vi "ArmRecoverHomePosition.vi"(0 "ArmRecoveryParameters In":T23, 1 "ArmRecoveryOffsets":T24, 2 "RobotConfig":T2={"Motors"={"DriveRightPrimary"={"CAN Address"=1, "Invert"=FALSE, "InvertSensor"=FALSE, "Unit Conversion Factor"=0.0, "Brake Mode"=enum."Override to Brake", "Reverse Limt Switch Mode"=enum."Normally Closed", "Forward Limt Swith Mode"=enum."Normally Closed", "PWM Channel"=enum."Invalid", "Motor Controller Type"=enum."Talon SRX", "Peak Current (A)"=0, "Continuos Current (A)"=0, "Peak Duration (ms)"=0, "Current Limit Enable"=FALSE}, "DriveRightSecondary"={"CAN Address"=2, "Invert"=FALSE, "InvertSensor"=FALSE, "Unit Conversion Factor"=0.0, "Brake Mode"=enum."Override to Brake", "Reverse Limt Switch Mode"=enum."Normally Closed", "Forward Limt Swith Mode"=enum."Normally Closed", "PWM Channel"=enum."Invalid", "Motor Controller Type"=enum."Talon SRX", "Peak Current (A)"=0, "Continuos Current (A)"=0, "Peak Duration (ms)"=0, "Current Limit Enable"=FALSE}, "DriveLeftPrimary"={"CAN Address"=3, "Invert"=FALSE, "InvertSensor"=FALSE, "Unit Conversion Factor"=0.0, "Brake Mode"=enum."Override to Brake", "Reverse Limt Switch Mode"=enum."Normally Closed", "Forward Limt Swith Mode"=enum."Normally Closed", "PWM Channel"=enum."Invalid", "Motor Controller Type"=enum."Talon SRX", "Peak Current (A)"=0, "Continuos Current (A)"=0, "Peak Duration (ms)"=0, "Current Limit Enable"=FALSE}, "DriveLeftSecondary"={"CAN Address"=4, "Invert"=FALSE, "InvertSensor"=FALSE, "Unit Conversion Factor"=0.0, "Brake Mode"=enum."Override to Brake", "Reverse Limt Switch Mode"=enum."Normally Closed", "Forward Limt Swith Mode"=enum."Normally Closed", "PWM Channel"=enum."Invalid", "Motor Controller Type"=enum."Talon SRX", "Peak Current (A)"=0, "Continuos Current (A)"=0, "Peak Duration (ms)"=0, "Current Limit Enable"=FALSE}, "RearClimb"={"CAN Address"=8, "Invert"=FALSE, "InvertSensor"=FALSE, "Unit Conversion Factor"=0.0, "Brake Mode"=enum."Override to Brake", "Reverse Limt Switch Mode"=enum."Normally Closed", "Forward Limt Swith Mode"=enum."Normally Closed", "PWM Channel"=enum."Invalid", "Motor Controller Type"=enum."Talon SRX", "Peak Current (A)"=0, "Continuos Current (A)"=0, "Peak Duration (ms)"=0, "Current Limit Enable"=FALSE}, "Front Climb"={"CAN Address"=7, "Invert"=FALSE, "InvertSensor"=FALSE, "Unit Conversion Factor"=0.0, "Brake Mode"=enum."Override to Brake", "Reverse Limt Switch Mode"=enum."Normally Closed", "Forward Limt Swith Mode"=enum."Normally Closed", "PWM Channel"=enum."Invalid", "Motor Controller Type"=enum."Talon SRX", "Peak Current (A)"=0, "Continuos Current (A)"=0, "Peak Duration (ms)"=0, "Current Limit Enable"=FALSE}, "Climb Drive"={"CAN Address"=5, "Invert"=FALSE, "InvertSensor"=FALSE, "Unit Conversion Factor"=0.0, "Brake Mode"=enum."Override to Brake", "Reverse Limt Switch Mode"=enum."Normally Closed", "Forward Limt Swith Mode"=enum."Normally Closed", "PWM Channel"=enum."Invalid", "Motor Controller Type"=enum."Talon SRX", "Peak Current (A)"=0, "Continuos Current (A)"=0, "Peak Duration (ms)"=0, "Current Limit Enable"=FALSE}, "Shoulder1"={"CAN Address"=6, "Invert"=FALSE, "InvertSensor"=FALSE, "Unit Conversion Factor"=0.0, "Brake Mode"=enum."Override to Brake", "Reverse Limt Switch Mode"=enum."Normally Closed", "Forward Limt Swith Mode"=enum."Normally Closed", "PWM Channel"=enum."Invalid", "Motor Controller Type"=enum."Talon SRX", "Peak Current (A)"=0, "Continuos Current (A)"=0, "Peak Duration (ms)"=0, "Current Limit Enable"=FALSE}, "Shoulder2"={"CAN Address"=9, "Invert"=FALSE, "InvertSensor"=FALSE, "Unit Conversion Factor"=0.0, "Brake Mode"=enum."Override to Brake", "Reverse Limt Switch Mode"=enum."Normally Closed", "Forward Limt Swith Mode"=enum."Normally Closed", "PWM Channel"=enum."Invalid", "Motor Controller Type"=enum."Talon SRX", "Peak Current (A)"=0, "Continuos Current (A)"=0, "Peak Duration (ms)"=0, "Current Limit Enable"=FALSE}, "Wrist"={"CAN Address"=10, "Invert"=FALSE, "InvertSensor"=FALSE, "Unit Conversion Factor"=0.0, "Brake Mode"=enum."Override to Brake", "Reverse Limt Switch Mode"=enum."Disabled", "Forward Limt Swith Mode"=enum."Disabled", "PWM Channel"=enum."Invalid", "Motor Controller Type"=enum."Talon SRX", "Peak Current (A)"=0, "Continuos Current (A)"=0, "Peak Duration (ms)"=0, "Current Limit Enable"=FALSE}, "Extension"={"CAN Address"=11, "Invert"=FALSE, "InvertSensor"=FALSE, "Unit Conversion Factor"=0.0, "Brake Mode"=enum."Override to Brake", "Reverse Limt Switch Mode"=enum."Disabled", "Forward Limt Swith Mode"=enum."Disabled", "PWM Channel"=enum."Invalid", "Motor Controller Type"=enum."Talon SRX", "Peak Current (A)"=0, "Continuos Current (A)"=0, "Peak Duration (ms)"=0, "Current Limit Enable"=FALSE}, "CargoIntake"={"CAN Address"=11, "Invert"=FALSE, "InvertSensor"=FALSE, "Unit Conversion Factor"=0.0, "Brake Mode"=enum."Override to Brake", "Reverse Limt Switch Mode"=enum."Disabled", "Forward Limt Swith Mode"=enum."Disabled", "PWM Channel"=enum."Invalid", "Motor Controller Type"=enum."Talon SRX", "Peak Current (A)"=0, "Continuos Current (A)"=0, "Peak Duration (ms)"=0, "Current Limit Enable"=FALSE}, "Intake2"={"CAN Address"=11, "Invert"=FALSE, "InvertSensor"=FALSE, "Unit Conversion Factor"=0.0, "Brake Mode"=enum."Override to Brake", "Reverse Limt Switch Mode"=enum."Disabled", "Forward Limt Swith Mode"=enum."Disabled", "PWM Channel"=enum."Invalid", "Motor Controller Type"=enum."Talon SRX", "Peak Current (A)"=0, "Continuos Current (A)"=0, "Peak Duration (ms)"=0, "Current Limit Enable"=FALSE}}, "Sensors"={"IMU"={"Yaw Axis"=enum."Z", "SPI Bus"=enum."SPI MXP", "AHRS Algorithm"=enum."Complementary", "Calibration Time (s)"=3.0, "Calibrate On Open"=TRUE}, "HomingButton"={"DIOChannel"=enum."DIO 0", "Active Low"=FALSE}, "HomingLED_Green"={"DIOChannel"=enum."DIO 0", "Active Low"=FALSE}, "HomingLED_Yellow"={"DIOChannel"=enum."DIO 0", "Active Low"=FALSE}, "HomingLED_Red"={"DIOChannel"=enum."DIO 0", "Active Low"=FALSE}}, "PID"={"FrontClimb"={"P"=0.0, "I"=0.0, "D"=0.0, "F"=0.0, "IZone"=0.0}, "RearClimb"={"P"=0.0, "I"=0.0, "D"=0.0, "F"=0.0, "IZone"=0.0}, "ArmShoulder"={"P"=0.0, "I"=0.0, "D"=0.0, "F"=0.0, "IZone"=0.0}, "ArmExtend"={"P"=0.0, "I"=0.0, "D"=0.0, "F"=0.0, "IZone"=0.0}, "ArmWrist"={"P"=0.0, "I"=0.0, "D"=0.0, "F"=0.0, "IZone"=0.0}}, "Solenoids"={" Shifter"={"SolenoidChannel"=enum."Solenoid 3", "Invert"=FALSE}, "Hatch Grip"={"SolenoidChannel"=enum."Solenoid 0", "Invert"=FALSE}, "Hatch Extend"={"SolenoidChannel"=enum."Solenoid 0", "Invert"=FALSE}, "Manipulator Slide"={"SolenoidChannel"=enum."Solenoid 0", "Invert"=FALSE}, "Hatch Floor Intake"={"SolenoidChannel"=enum."Solenoid 0", "Invert"=FALSE}}, "Enable Compressor"=TRUE, "MotionMagic"={"FrontClimbExtend"={"CruiseVelocity"=0, "Acceleration"=0}, "RearClimbExtend"={"CruiseVelocity"=0, "Acceleration"=0}, "FrontClimbRetract"={"CruiseVelocity"=0, "Acceleration"=0}, "RearClimbRetract"={"CruiseVelocity"=0, "Acceleration"=0}}, "RobotDimensions"={"Length (in)"=0.0, "Shoulder Height (in)"=0.0, "Frame Height (in)"=0.0, "Arm Center to Front of Robot (in)"=0.0, "Arm Min Extension (in)"=0.0, "Arm Max Extension (in)"=0.0, "Cargo Intake Loop Length (in)"=0.0, "Cargo Intake Loop Width (in)"=0.0, "Cargo Intake Loop Offset (in)"=0.0, "Cargo Intake Loop Angle (rad)"=0.0}, "Arm Home Position"={"Radius (in)"=0.0, "ShoulderAngle (rad)"=0.0, "WristAngle (rad)"=0.0}, "Climb Home Position"={"Back Climb"=0.0, "Front Climb"=0.0}, "Climb Positions"={"Retract"=0.0, "Level 2"=0.0, "Level 3"=0.0}}, 3 "RobotMotors":T19={"DriveRightPrimary"={"DeviceStatus"={"status"=FALSE, "code"=0, "source"=""}, "Type"=enum."PWM", "PWM"={"PWM Channel"=enum."PWM 1", "DeadBand"={"Name"="", "maxPositivePwm"=0, "minPositivePwm"=0, "centerPwm"=0, "maxNegativePwm"=0, "minNegativePwm"=0, "angularRange"=0}}, "CAN"={"Device Number"=0, "SetOutput VI Ref"=variant(enum8{"Percent VBus", "Current", "Speed", "Position", "Voltage"} enum."Percent VBus"), "GetOutput VI Ref"=variant(refnum<k1> refnum), "Enable VI Ref"=variant(dbl 12.0), "Disable VI Ref"=variant(enum8{"Percent VBus", "Speed", "Position", "Slave", "Unchanged / Invalid", "Voltage Compensation", "Current", "Motion Profile"} enum."Percent VBus"), "Data"=variant}, "Invert"=FALSE, "DIO PWM"={"PWM \"Enable\" Channel"=enum."Invalid", "DIOChannel"=enum."Invalid", "PWM Rate"=0.0}}, "DriveRightSecondary"={"DeviceStatus"={"status"=FALSE, "code"=0, "source"=""}, "Type"=enum."PWM", "PWM"={"PWM Channel"=enum."PWM 1", "DeadBand"={"Name"="", "maxPositivePwm"=0, "minPositivePwm"=0, "centerPwm"=0, "maxNegativePwm"=0, "minNegativePwm"=0, "angularRange"=0}}, "CAN"={"Device Number"=0, "SetOutput VI Ref"=variant(enum8{"Percent VBus", "Current", "Speed", "Position", "Voltage"} enum."Percent VBus"), "GetOutput VI Ref"=variant(refnum<k1> refnum), "Enable VI Ref"=variant(dbl 12.0), "Disable VI Ref"=variant(enum8{"Percent VBus", "Speed", "Position", "Slave", "Unchanged / Invalid", "Voltage Compensation", "Current", "Motion Profile"} enum."Percent VBus"), "Data"=variant}, "Invert"=FALSE, "DIO PWM"={"PWM \"Enable\" Channel"=enum."Invalid", "DIOChannel"=enum."Invalid", "PWM Rate"=0.0}}, "DriveLeftPrimary"={"DeviceStatus"={"status"=FALSE, "code"=0, "source"=""}, "Type"=enum."PWM", "PWM"={"PWM Channel"=enum."PWM 1", "DeadBand"={"Name"="", "maxPositivePwm"=0, "minPositivePwm"=0, "centerPwm"=0, "maxNegativePwm"=0, "minNegativePwm"=0, "angularRange"=0}}, "CAN"={"Device Number"=0, "SetOutput VI Ref"=variant(enum8{"Percent VBus", "Current", "Speed", "Position", "Voltage"} enum."Percent VBus"), "GetOutput VI Ref"=variant(refnum<k1> refnum), "Enable VI Ref"=variant(dbl 12.0), "Disable VI Ref"=variant(enum8{"Percent VBus", "Speed", "Position", "Slave", "Unchanged / Invalid", "Voltage Compensation", "Current", "Motion Profile"} enum."Percent VBus"), "Data"=variant}, "Invert"=FALSE, "DIO PWM"={"PWM \"Enable\" Channel"=enum."Invalid", "DIOChannel"=enum."Invalid", "PWM Rate"=0.0}}, "DriveLeftSecondary"={"DeviceStatus"={"status"=FALSE, "code"=0, "source"=""}, "Type"=enum."PWM", "PWM"={"PWM Channel"=enum."PWM 1", "DeadBand"={"Name"="", "maxPositivePwm"=0, "minPositivePwm"=0, "centerPwm"=0, "maxNegativePwm"=0, "minNegativePwm"=0, "angularRange"=0}}, "CAN"={"Device Number"=0, "SetOutput VI Ref"=variant(enum8{"Percent VBus", "Current", "Speed", "Position", "Voltage"} enum."Percent VBus"), "GetOutput VI Ref"=variant(refnum<k1> refnum), "Enable VI Ref"=variant(dbl 12.0), "Disable VI Ref"=variant(enum8{"Percent VBus", "Speed", "Position", "Slave", "Unchanged / Invalid", "Voltage Compensation", "Current", "Motion Profile"} enum."Percent VBus"), "Data"=variant}, "Invert"=FALSE, "DIO PWM"={"PWM \"Enable\" Channel"=enum."Invalid", "DIOChannel"=enum."Invalid", "PWM Rate"=0.0}}, " RearClimb"={"DeviceStatus"={"status"=FALSE, "code"=0, "source"=""}, "Type"=enum."PWM", "PWM"={"PWM Channel"=enum."PWM 1", "DeadBand"={"Name"="", "maxPositivePwm"=0, "minPositivePwm"=0, "centerPwm"=0, "maxNegativePwm"=0, "minNegativePwm"=0, "angularRange"=0}}, "CAN"={"Device Number"=0, "SetOutput VI Ref"=variant(enum8{"Percent VBus", "Current", "Speed", "Position", "Voltage"} enum."Percent VBus"), "GetOutput VI Ref"=variant(refnum<k1> refnum), "Enable VI Ref"=variant(dbl 12.0), "Disable VI Ref"=variant(enum8{"Percent VBus", "Speed", "Position", "Slave", "Unchanged / Invalid", "Voltage Compensation", "Current", "Motion Profile"} enum."Percent VBus"), "Data"=variant}, "Invert"=FALSE, "DIO PWM"={"PWM \"Enable\" Channel"=enum."Invalid", "DIOChannel"=enum."Invalid", "PWM Rate"=0.0}}, "FrontClimb"={"DeviceStatus"={"status"=FALSE, "code"=0, "source"=""}, "Type"=enum."PWM", "PWM"={"PWM Channel"=enum."PWM 1", "DeadBand"={"Name"="", "maxPositivePwm"=0, "minPositivePwm"=0, "centerPwm"=0, "maxNegativePwm"=0, "minNegativePwm"=0, "angularRange"=0}}, "CAN"={"Device Number"=0, "SetOutput VI Ref"=variant(enum8{"Percent VBus", "Current", "Speed", "Position", "Voltage"} enum."Percent VBus"), "GetOutput VI Ref"=variant(refnum<k1> refnum), "Enable VI Ref"=variant(dbl 12.0), "Disable VI Ref"=variant(enum8{"Percent VBus", "Speed", "Position", "Slave", "Unchanged / Invalid", "Voltage Compensation", "Current", "Motion Profile"} enum."Percent VBus"), "Data"=variant}, "Invert"=FALSE, "DIO PWM"={"PWM \"Enable\" Channel"=enum."Invalid", "DIOChannel"=enum."Invalid", "PWM Rate"=0.0}}, "ClimbDrive"={"DeviceStatus"={"status"=FALSE, "code"=0, "source"=""}, "Type"=enum."PWM", "PWM"={"PWM Channel"=enum."PWM 1", "DeadBand"={"Name"="", "maxPositivePwm"=0, "minPositivePwm"=0, "centerPwm"=0, "maxNegativePwm"=0, "minNegativePwm"=0, "angularRange"=0}}, "CAN"={"Device Number"=0, "SetOutput VI Ref"=variant(enum8{"Percent VBus", "Current", "Speed", "Position", "Voltage"} enum."Percent VBus"), "GetOutput VI Ref"=variant(refnum<k1> refnum), "Enable VI Ref"=variant(dbl 12.0), "Disable VI Ref"=variant(enum8{"Percent VBus", "Speed", "Position", "Slave", "Unchanged / Invalid", "Voltage Compensation", "Current", "Motion Profile"} enum."Percent VBus"), "Data"=variant}, "Invert"=FALSE, "DIO PWM"={"PWM \"Enable\" Channel"=enum."Invalid", "DIOChannel"=enum."Invalid", "PWM Rate"=0.0}}, "Shoulder2"={"DeviceStatus"={"status"=FALSE, "code"=0, "source"=""}, "Type"=enum."PWM", "PWM"={"PWM Channel"=enum."PWM 1", "DeadBand"={"Name"="", "maxPositivePwm"=0, "minPositivePwm"=0, "centerPwm"=0, "maxNegativePwm"=0, "minNegativePwm"=0, "angularRange"=0}}, "CAN"={"Device Number"=0, "SetOutput VI Ref"=variant(enum8{"Percent VBus", "Current", "Speed", "Position", "Voltage"} enum."Percent VBus"), "GetOutput VI Ref"=variant(refnum<k1> refnum), "Enable VI Ref"=variant(dbl 12.0), "Disable VI Ref"=variant(enum8{"Percent VBus", "Speed", "Position", "Slave", "Unchanged / Invalid", "Voltage Compensation", "Current", "Motion Profile"} enum."Percent VBus"), "Data"=variant}, "Invert"=FALSE, "DIO PWM"={"PWM \"Enable\" Channel"=enum."Invalid", "DIOChannel"=enum."Invalid", "PWM Rate"=0.0}}, "Shoulder1 "={"DeviceStatus"={"status"=FALSE, "code"=0, "source"=""}, "Type"=enum."PWM", "PWM"={"PWM Channel"=enum."PWM 1", "DeadBand"={"Name"="", "maxPositivePwm"=0, "minPositivePwm"=0, "centerPwm"=0, "maxNegativePwm"=0, "minNegativePwm"=0, "angularRange"=0}}, "CAN"={"Device Number"=0, "SetOutput VI Ref"=variant(enum8{"Percent VBus", "Current", "Speed", "Position", "Voltage"} enum."Percent VBus"), "GetOutput VI Ref"=variant(refnum<k1> refnum), "Enable VI Ref"=variant(dbl 12.0), "Disable VI Ref"=variant(enum8{"Percent VBus", "Speed", "Position", "Slave", "Unchanged / Invalid", "Voltage Compensation", "Current", "Motion Profile"} enum."Percent VBus"), "Data"=variant}, "Invert"=FALSE, "DIO PWM"={"PWM \"Enable\" Channel"=enum."Invalid", "DIOChannel"=enum."Invalid", "PWM Rate"=0.0}}, "Wrist"={"DeviceStatus"={"status"=FALSE, "code"=0, "source"=""}, "Type"=enum."PWM", "PWM"={"PWM Channel"=enum."PWM 1", "DeadBand"={"Name"="", "maxPositivePwm"=0, "minPositivePwm"=0, "centerPwm"=0, "maxNegativePwm"=0, "minNegativePwm"=0, "angularRange"=0}}, "CAN"={"Device Number"=0, "SetOutput VI Ref"=variant(enum8{"Percent VBus", "Current", "Speed", "Position", "Voltage"} enum."Percent VBus"), "GetOutput VI Ref"=variant(refnum<k1> refnum), "Enable VI Ref"=variant(dbl 12.0), "Disable VI Ref"=variant(enum8{"Percent VBus", "Speed", "Position", "Slave", "Unchanged / Invalid", "Voltage Compensation", "Current", "Motion Profile"} enum."Percent VBus"), "Data"=variant}, "Invert"=FALSE, "DIO PWM"={"PWM \"Enable\" Channel"=enum."Invalid", "DIOChannel"=enum."Invalid", "PWM Rate"=0.0}}, "Extension"={"DeviceStatus"={"status"=FALSE, "code"=0, "source"=""}, "Type"=enum."PWM", "PWM"={"PWM Channel"=enum."PWM 1", "DeadBand"={"Name"="", "maxPositivePwm"=0, "minPositivePwm"=0, "centerPwm"=0, "maxNegativePwm"=0, "minNegativePwm"=0, "angularRange"=0}}, "CAN"={"Device Number"=0, "SetOutput VI Ref"=variant(enum8{"Percent VBus", "Current", "Speed", "Position", "Voltage"} enum."Percent VBus"), "GetOutput VI Ref"=variant(refnum<k1> refnum), "Enable VI Ref"=variant(dbl 12.0), "Disable VI Ref"=variant(enum8{"Percent VBus", "Speed", "Position", "Slave", "Unchanged / Invalid", "Voltage Compensation", "Current", "Motion Profile"} enum."Percent VBus"), "Data"=variant}, "Invert"=FALSE, "DIO PWM"={"PWM \"Enable\" Channel"=enum."Invalid", "DIOChannel"=enum."Invalid", "PWM Rate"=0.0}}, "CargoIntake"={"DeviceStatus"={"status"=FALSE, "code"=0, "source"=""}, "Type"=enum."PWM", "PWM"={"PWM Channel"=enum."PWM 1", "DeadBand"={"Name"="", "maxPositivePwm"=0, "minPositivePwm"=0, "centerPwm"=0, "maxNegativePwm"=0, "minNegativePwm"=0, "angularRange"=0}}, "CAN"={"Device Number"=0, "SetOutput VI Ref"=variant(enum8{"Percent VBus", "Current", "Speed", "Position", "Voltage"} enum."Percent VBus"), "GetOutput VI Ref"=variant(refnum<k1> refnum), "Enable VI Ref"=variant(dbl 12.0), "Disable VI Ref"=variant(enum8{"Percent VBus", "Speed", "Position", "Slave", "Unchanged / Invalid", "Voltage Compensation", "Current", "Motion Profile"} enum."Percent VBus"), "Data"=variant}, "Invert"=FALSE, "DIO PWM"={"PWM \"Enable\" Channel"=enum."Invalid", "DIOChannel"=enum."Invalid", "PWM Rate"=0.0}}, "Intake2"={"DeviceStatus"={"status"=FALSE, "code"=0, "source"=""}, "Type"=enum."PWM", "PWM"={"PWM Channel"=enum."PWM 1", "DeadBand"={"Name"="", "maxPositivePwm"=0, "minPositivePwm"=0, "centerPwm"=0, "maxNegativePwm"=0, "minNegativePwm"=0, "angularRange"=0}}, "CAN"={"Device Number"=0, "SetOutput VI Ref"=variant(enum8{"Percent VBus", "Current", "Speed", "Position", "Voltage"} enum."Percent VBus"), "GetOutput VI Ref"=variant(refnum<k1> refnum), "Enable VI Ref"=variant(dbl 12.0), "Disable VI Ref"=variant(enum8{"Percent VBus", "Speed", "Position", "Slave", "Unchanged / Invalid", "Voltage Compensation", "Current", "Motion Profile"} enum."Percent VBus"), "Data"=variant}, "Invert"=FALSE, "DIO PWM"={"PWM \"Enable\" Channel"=enum."Invalid", "DIOChannel"=enum."Invalid", "PWM Rate"=0.0}}}, 5 "ArmHomingStateIn":T26=enum."homing failed", 9 "ArmPositionValidityIn":T27, 11 "ArmHomingValidityIn":T25=enum."Invalid", 12 "RecoveredIn":bool) -> (4 "ArmRecoveryParameters Out":T23, 6 "ArmHomingStateOut":T26=enum."homing failed", 10 "ArmPositionValidityOut":T27, 14 "RecoveredOut":bool, 15 "ArmHomingValidityOut":T25=enum."Invalid")   [LabVIEW 2018]
uses:
  TypeDefs/ArmPositionComponentValidity.ctl
  TypeDefs/ArmPositionRecoveryParams.ctl
  TypeDefs/ArmHomingState.ctl
  TypeDefs/ArmHomingValidity.ctl
  TypeDefs/ArmPositionRecoveryOffsets.ctl
  TypeDefs/RobotComponents/RobotMotors.ctl
  <vilib>/Rock Robotics/WPI/MotorControl/WPI_MotorControlDeviceRef.ctl
  <vilib>/Rock Robotics/WPI/MotorControl/WPI_MotorControlType.ctl
  <vilib>/Rock Robotics/SystemInterfaces/DIO/FPGA_DIOPWMChannel.ctl
  <vilib>/Rock Robotics/WPI/PWM/WPI_PWMDeadband.ctl
  <vilib>/Rock Robotics/SystemInterfaces/DIO/FPGA_DIOChannel.ctl
  TypeDefs/ConfigComponents/Config_Robot.ctl
  ArgosLib/Config/ConfigComponents/TypeDefs/Config_Motor.ctl
  <vilib>/Rock Robotics/WPI/ThirdParty/Phoenix-LabVIEW/Motor Controller/Controls/CTRE_Phoenix_MotorControl_NeutralMode.ctl
  <vilib>/Rock Robotics/WPI/ThirdParty/Phoenix-LabVIEW/Motor Controller/Controls/CTRE_Phoenix_MotorControl_LimitSwitchNormal.ctl
  ArgosLib/Config/ConfigComponents/TypeDefs/Config_MotorCtrlType.ctl
  ArgosLib/Config/ConfigComponents/TypeDefs/Config_IMU.ctl
  <vilib>/Rock Robotics/SystemInterfaces/spilib/spi_bus.ctl
  ArgosLib/Config/ConfigComponents/TypeDefs/Config_DigitalIO.ctl
  ArgosLib/Config/ConfigComponents/TypeDefs/Config_PIDParams.ctl
  ArgosLib/Config/ConfigComponents/TypeDefs/Config_SingleSolenoid.ctl
  <vilib>/Rock Robotics/WPI/Solenoid/WPI_SolenoidChannel.ctl
  ArgosLib/Config/ConfigComponents/TypeDefs/Config_MotionMagicParams.ctl
  TypeDefs/ConfigComponents/Config_Dimensions.ctl
  TypeDefs/ArmCoordinate.ctl
  Climber/TypeDefs/ClimberPositionHeights.ctl
  ArgosLib/ArgosLib.lvlib
panel:
  out "WristRecover":T1
  out "ExtensionRecover":T1
  out "ShoulderRecover":T1
  out "LatestComponentQuadPositions":T23
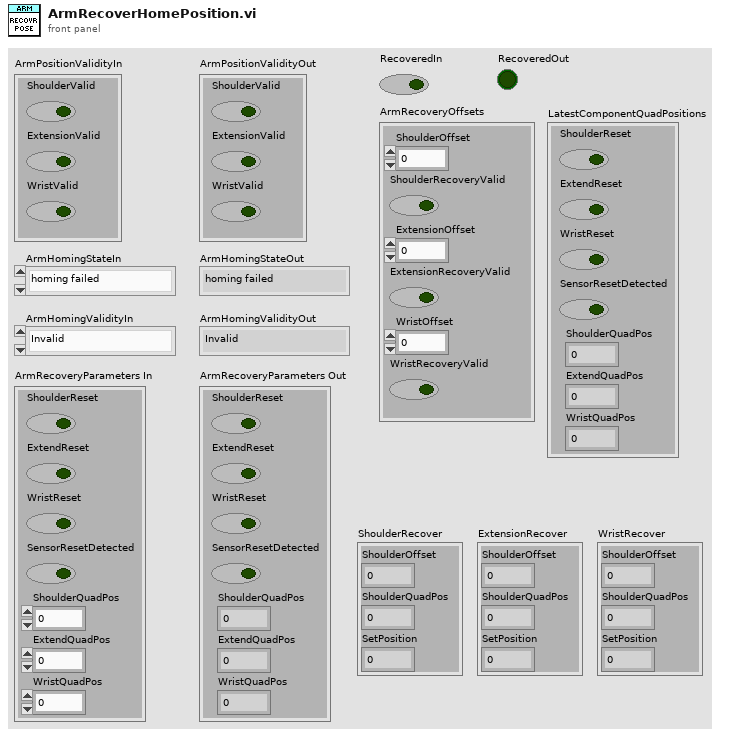
[diagram p1: front panel]
types:
  T1 = cluster{"ShoulderOffset":i32, "ShoulderQuadPos":i32, "SetPosition":i32}
  T2 = typedef "Config_Robot.ctl" = cluster{"Motors":cluster{"DriveRightPrimary":T3, "DriveRightSecondary":T3, "DriveLeftPrimary":T3, "DriveLeftSecondary":T3, "RearClimb":T3, "Front Climb":T3, "Climb Drive":T3, "Shoulder1":T3, "Shoulder2":T3, "Wrist":T3, "Extension":T3, "CargoIntake":T3, "Intake2":T3}, "Sensors":cluster{"IMU":T8, "HomingButton":T10, "HomingLED_Green":T10, "HomingLED_Yellow":T10, "HomingLED_Red":T10}, "PID":cluster{"FrontClimb":T12, "RearClimb":T12, "ArmShoulder":T12, "ArmExtend":T12, "ArmWrist":T12}, "Solenoids":cluster{" Shifter":T13, "Hatch Grip":T13, "Hatch Extend":T13, "Manipulator Slide":T13, "Hatch Floor Intake":T13}, "Enable Compressor":bool, "MotionMagic":cluster{"FrontClimbExtend":T15, "RearClimbExtend":T15, "FrontClimbRetract":T15, "RearClimbRetract":T15}, "RobotDimensions":T16, "Arm Home Position":T17, "Climb Home Position":cluster{"Back Climb":dbl, "Front Climb":dbl}, "Climb Positions":T18}
  T3 = typedef "ArgosLib.lvlib/Config_Motor.ctl" = cluster{"CAN Address":u8, "Invert":bool, "InvertSensor":bool, "Unit Conversion Factor":dbl, "Brake Mode":T4, "Reverse Limt Switch Mode":T5, "Forward Limt Swith Mode":T5, "PWM Channel":T6, "Motor Controller Type":T7, "Peak Current (A)":i32, "Continuos Current (A)":i32, "Peak Duration (ms)":i32, "Current Limit Enable":bool}
  T4 = typedef "CTRE_Phoenix_MotorControl_NeutralMode.ctl" = enum8{"EEPROMSetting", "Override to Coast", "Override to Brake"}
  T5 = typedef "CTRE_Phoenix_MotorControl_LimitSwitchNormal.ctl" = enum16{"Normally Open", "Normally Closed", "Disabled"}
  T6 = typedef "FPGA_DIOPWMChannel.ctl" = enum8{"PWM 0", "PWM 1", "PWM 2", "PWM 3", "PWM 4", "PWM 5", "PWM 6", "PWM 7", "PWM 8", "PWM 9", "PWM MXP 0", "PWM MXP 1", "PWM MXP 2", "PWM MXP 3", "PWM MXP 4", "PWM MXP 5", "PWM MXP 6", "PWM MXP 7", "PWM MXP 8", "PWM MXP 9", "Invalid"}
  T7 = typedef "ArgosLib.lvlib/Config_MotorCtrlType.ctl" = enum16{"Disabled", "Talon SRX", "Talon SR"}
  T8 = typedef "ArgosLib.lvlib/Config_IMU.ctl" = cluster{"Yaw Axis":enum16{"X", "Y", "Z"}, "SPI Bus":T9, "AHRS Algorithm":enum16{"Complementary", "Madgwick"}, "Calibration Time (s)":dbl, "Calibrate On Open":bool}
  T9 = typedef "spi_bus.ctl" = enum16{"SPI On-Board, CS0", "SPI On-Board, CS1", "SPI On-Board, CS2", "SPI On-Board, CS3", "SPI MXP", "Invalid"}
  T10 = typedef "ArgosLib.lvlib/Config_DigitalIO.ctl" = cluster{"DIOChannel":T11, "Active Low":bool}
  T11 = typedef "FPGA_DIOChannel.ctl" = enum8{"DIO 0", "DIO 1", "DIO 2", "DIO 3", "DIO 4", "DIO 5", "DIO 6", "DIO 7", "DIO 8", "DIO 9", "DIO MXP 0", "DIO MXP 1", "DIO MXP 2", "DIO MXP 3", "DIO MXP 4", "DIO MXP 5", "DIO MXP 6", "DIO MXP 7", "DIO MXP 8", "DIO MXP 9", "DIO MXP 10", "DIO MXP 11", "DIO MXP 12", "DIO MXP 13", "DIO MXP 14", "DIO MXP 15", "SPI Port CS1", "SPI Port CS2", "SPI Port CS3", "SPI Port MISO", "SPI Port MOSI", "Invalid"}
  T12 = typedef "ArgosLib.lvlib/Config_PIDParams.ctl" = cluster{"P":dbl, "I":dbl, "D":dbl, "F":dbl, "IZone":dbl}
  T13 = typedef "ArgosLib.lvlib/Config_SingleSolenoid.ctl" = cluster{"SolenoidChannel":T14, "Invert":bool}
  T14 = typedef "WPI_SolenoidChannel.ctl" = enum8{"Solenoid 0", "Solenoid 1", "Solenoid 2", "Solenoid 3", "Solenoid 4", "Solenoid 5", "Solenoid 6", "Solenoid 7", "Invalid"}
  T15 = typedef "Config_MotionMagicParams.ctl" = cluster{"CruiseVelocity":i32, "Acceleration":i32}
  T16 = typedef "Config_Dimensions.ctl" = cluster{"Length (in)":dbl, "Shoulder Height (in)":dbl, "Frame Height (in)":dbl, "Arm Center to Front of Robot (in)":dbl, "Arm Min Extension (in)":dbl, "Arm Max Extension (in)":dbl, "Cargo Intake Loop Length (in)":dbl, "Cargo Intake Loop Width (in)":dbl, "Cargo Intake Loop Offset (in)":dbl, "Cargo Intake Loop Angle (rad)":dbl}
  T17 = typedef "ArmCoordinate.ctl" = cluster{"Radius (in)":dbl, "ShoulderAngle (rad)":dbl, "WristAngle (rad)":dbl}
  T18 = typedef "ClimberPositionHeights.ctl" = cluster{"Retract":dbl, "Level 2":dbl, "Level 3":dbl}
  T19 = typedef "RobotMotors.ctl" = cluster{"DriveRightPrimary":T20, "DriveRightSecondary":T20, "DriveLeftPrimary":T20, "DriveLeftSecondary":T20, " RearClimb":T20, "FrontClimb":T20, "ClimbDrive":T20, "Shoulder2":T20, "Shoulder1 ":T20, "Wrist":T20, "Extension":T20, "CargoIntake":T20, "Intake2":T20}
  T20 = typedef "WPI_MotorControlDeviceRef.ctl" = cluster{"DeviceStatus":errorcluster, "Type":T21, "PWM":cluster{"PWM Channel":T6, "DeadBand":T22}, "CAN":cluster{"Device Number":u8, "SetOutput VI Ref":variant, "GetOutput VI Ref":variant, "Enable VI Ref":variant, "Disable VI Ref":variant, "Data":variant}, "Invert":bool, "DIO PWM":cluster{"PWM \"Enable\" Channel":T6, "DIOChannel":T11, "PWM Rate":dbl}}
  T21 = typedef "WPI_MotorControlType.ctl" = enum16{"PWM", "CAN", "DIO PWM"}
  T22 = typedef "WPI_PWMDeadband.ctl" = cluster{"Name":string, "maxPositivePwm":i32, "minPositivePwm":i32, "centerPwm":i32, "maxNegativePwm":i32, "minNegativePwm":i32, "angularRange":u16}
  T23 = typedef "ArmPositionRecoveryParams.ctl" = cluster{"ShoulderReset":bool, "ExtendReset":bool, "WristReset":bool, "SensorResetDetected":bool, "ShoulderQuadPos":i32, "ExtendQuadPos":i32, "WristQuadPos":i32}
  T24 = typedef "ArmPositionRecoveryOffsets.ctl" = cluster{"ShoulderOffset":i32, "ShoulderRecoveryValid":bool, "ExtensionOffset":i32, "ExtensionRecoveryValid":bool, "WristOffset":i32, "WristRecoveryValid":bool}
  T25 = typedef "ArmHomingValidity.ctl" = enum16{"Incomplete", "Valid", "Invalid"}
  T26 = typedef "ArmHomingState.ctl" = enum16{"ready", "homing in progress", "homing complete ", "homing failed"}
  T27 = typedef "ArmPositionComponentValidity.ctl" = cluster{"ShoulderValid":bool, "ExtensionValid":bool, "WristValid":bool}
  T28 = cluster{"ExtensionOffset":i32, "ExtendQuadPos":i32, "SetPosition":i32}
  T29 = cluster{"WristOffset":i32, "WristQuadPos":i32, "SetPosition":i32}
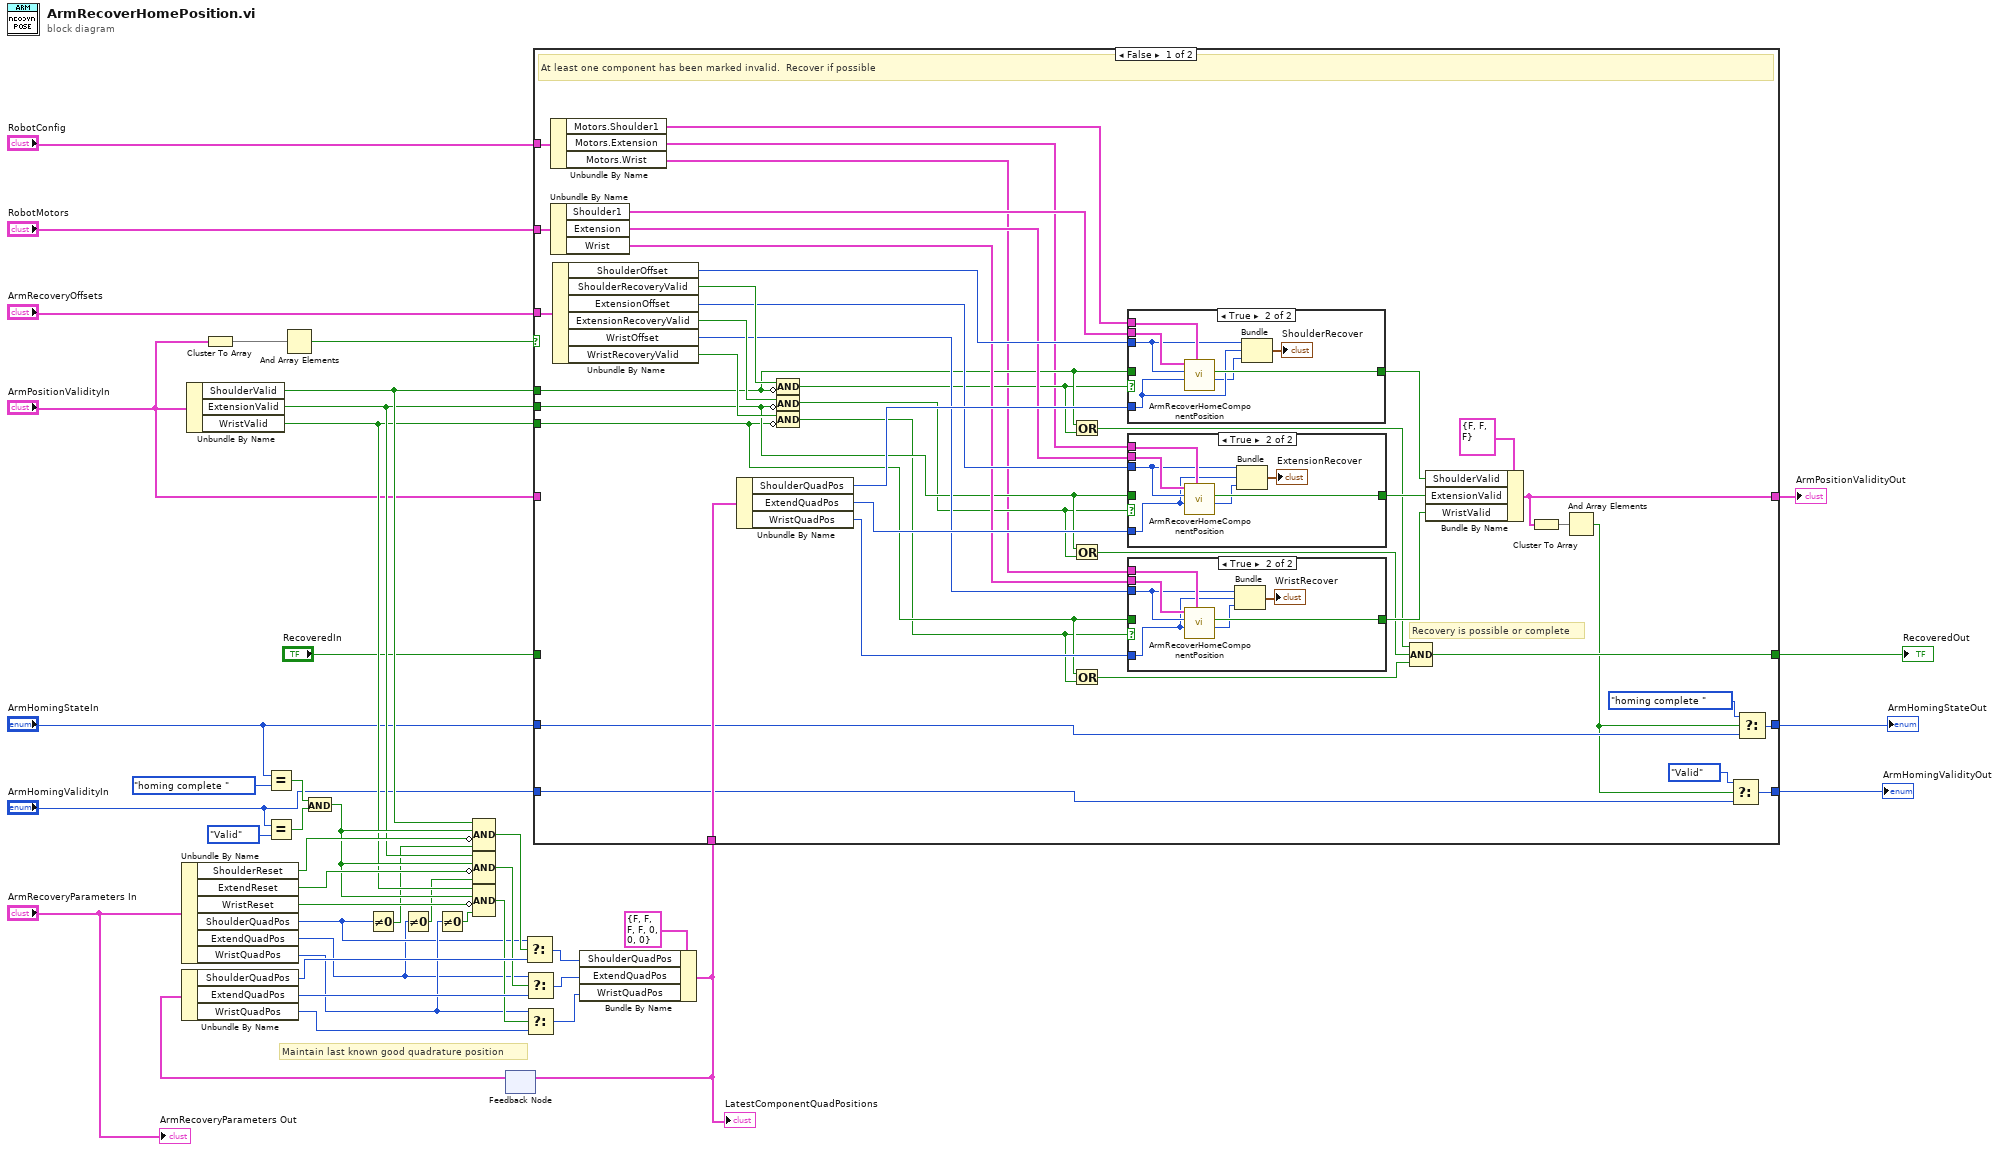
[diagram p0: block diagram]
diagram:
  # "Maintain last known good quadrature position"
  n1 = Unbundle By Name("ArmRecoveryParameters In") -> ("ShoulderReset"=w31:bool, "ExtendReset"=w30:bool, "WristReset"=w28:bool, "ShoulderQuadPos"=w5:i32, "ExtendQuadPos"=w4:i32, "WristQuadPos"=w6:i32)
  n2 = Unbundle By Name("ArmPositionValidityIn") -> ("ShoulderValid"=w21:bool, "ExtensionValid"=w20:bool, "WristValid"=w18:bool)
  n3 = Cluster To Array(cluster="ArmPositionValidityIn") -> (array=w17:bool[])
  n4 = Equal?(x="ArmHomingStateIn", y=ArmHomingState."homing complete ") -> (x = y?=w33:bool)
  n5 = Equal?(x="ArmHomingValidityIn", y=ArmHomingValidity."Valid") -> (x = y?=w32:bool)
  n6 = And Array Elements(Boolean array=w17) -> (logical AND=w16:bool)
  n7 = And(x=w33, y=w32) -> (x .and. y?=w29:bool)
  n8 = Not Equal To 0?(x=w5) -> (x != 0?=w2:bool)
  n9 = Not Equal To 0?(x=w4) -> (x != 0?=w3:bool)
  n10 = Not Equal To 0?(x=w6) -> (x != 0?=w7:bool)
  n11 = Compound Arithmetic op=AND(w21, w29, invert w31, w2) -> (w27:bool)
  n12 = Compound Arithmetic op=AND(w20, w29, invert w30, w3) -> (w26:bool)
  n13 = Compound Arithmetic op=AND(w18, w29, invert w28, w7) -> (w25:bool)
  n14 = feedback #1() -> (w40:T23)  [unwired: 1 in]
  n15 = Unbundle By Name(w40) -> ("ShoulderQuadPos"=w37:i32, "ExtendQuadPos"=w38:i32, "WristQuadPos"=w39:i32)
  n16 = Select(t=w5, s=w27, f=w37) -> (s? t:f=w36:i32)
  n17 = Select(t=w4, s=w26, f=w38) -> (s? t:f=w35:i32)
  n18 = Select(t=w6, s=w25, f=w39) -> (s? t:f=w34:i32)
  n19 = Bundle By Name(cluster=T23 {"ShoulderReset"=FALSE, "ExtendReset"=FALSE, "WristReset"=FALSE, "SensorResetDetected"=FALSE, "ShoulderQuadPos"=0, "ExtendQuadPos"=0, "WristQuadPos"=0} ("ArmRecoveryParameters In"), "ShoulderQuadPos"=w36, "ExtendQuadPos"=w35, "WristQuadPos"=w34) -> (w22:T23)
  "LatestComponentQuadPositions" <- w22
  n20 = feedback-in #1(w22) -> ()
  n21 = case shown="False" w16 {
    tunnel: "RobotMotors" -> [w85 _]
    tunnel: "ArmRecoveryOffsets" -> [w84 _]
    tunnel: w22 -> [w78 _]
    tunnel: w21 -> [w66 _]
    tunnel: w20 -> [w64 _]
    tunnel: [w56 w112] -> w19
    tunnel: w18 -> [w62 _]
    tunnel: [w57 w113] -> w15
    tunnel: "RecoveredIn" -> [_ w113]
    tunnel: "ArmPositionValidityIn" -> [_ w112]
    tunnel: "ArmHomingStateIn" -> [w52 w111]
    tunnel: "ArmHomingValidityIn" -> [w51 w110]
    tunnel: [w53 w111] -> w10
    tunnel: [w50 w110] -> w9
    tunnel: "RobotConfig" -> [w47 _]
    frame False {
      # "Recovery is possible or complete"
      # "At least one component has been marked invalid.  Recover if possible"
      n22 = Unbundle By Name(w47) -> ("Motors.Shoulder1"=w46:T3, "Motors.Extension"=w45:T3, "Motors.Wrist"=w44:T3)
      n23 = Unbundle By Name(w85) -> ("Shoulder1"=w80:T20, "Extension"=w76:T20, "Wrist"=w73:T20)
      n24 = Unbundle By Name(w84) -> ("ShoulderOffset"=w79:i32, "ShoulderRecoveryValid"=w83:bool, "ExtensionOffset"=w74:i32, "ExtensionRecoveryValid"=w82:bool, "WristOffset"=w72:i32, "WristRecoveryValid"=w81:bool)
      n25 = Unbundle By Name(w78) -> ("ShoulderQuadPos"=w77:i32, "ExtendQuadPos"=w75:i32, "WristQuadPos"=w71:i32)
      n26 = Compound Arithmetic op=AND(w83, invert w66) -> (w65:bool)
      n27 = Compound Arithmetic op=AND(w82, invert w64) -> (w63:bool)
      n28 = Compound Arithmetic op=AND(w81, invert w62) -> (w61:bool)
      n29 = Or(x=w66, y=w65) -> (x .or. y?=w60:bool)
      n30 = Or(x=w64, y=w63) -> (x .or. y?=w59:bool)
      n31 = Or(x=w62, y=w61) -> (x .or. y?=w58:bool)
      n32 = case shown="True" w65 {
        tunnel: w80 -> [_ w109]
        tunnel: w79 -> [_ w106]
        tunnel: w77 -> [_ w105]
        tunnel: [w102 w108] -> w69
        tunnel: w66 -> [w102 _]
        tunnel: w46 -> [_ w107]
        frame False {
        }
        frame True {
          n33 = call "ArmRecoverHomeComponentPosition.vi"("MotorConfig"=w107, "LatestQuadPosition"=w105, "AbsoluteOffset"=w106, "PhoenixMotorControlDevRefIn"=w109) -> ("SetPosition"=w104:i32, "Success"=w108:bool)  [unwired: 4 in, 2 out]
          n34 = Bundle("ShoulderOffset"=w106, "ShoulderQuadPos"=w105, "SetPosition"=w104) -> (→"ShoulderRecover":T1)  [unwired: 1 in]
        }
      }
      n35 = case shown="True" w63 {
        tunnel: w76 -> [_ w101]
        tunnel: w74 -> [_ w97]
        tunnel: w75 -> [_ w96]
        tunnel: [w94 w100] -> w68
        tunnel: w64 -> [w94 _]
        tunnel: w45 -> [_ w99]
        frame False {
        }
        frame True {
          n36 = call "ArmRecoverHomeComponentPosition.vi"("MotorConfig"=w99, "LatestQuadPosition"=w96, "AbsoluteOffset"=w97, "PhoenixMotorControlDevRefIn"=w101) -> ("SetPosition"=w95:i32, "Success"=w100:bool)  [unwired: 4 in, 2 out]
          n37 = Bundle("ExtensionOffset"=w97, "ExtendQuadPos"=w96, "SetPosition"=w95) -> (→"ExtensionRecover":T28)  [unwired: 1 in]
        }
      }
      n38 = case shown="True" w61 {
        tunnel: w73 -> [_ w93]
        tunnel: w72 -> [_ w89]
        tunnel: w71 -> [_ w88]
        tunnel: [w86 w92] -> w67
        tunnel: w62 -> [w86 _]
        tunnel: w44 -> [_ w91]
        frame False {
        }
        frame True {
          n39 = call "ArmRecoverHomeComponentPosition.vi"("MotorConfig"=w91, "LatestQuadPosition"=w88, "AbsoluteOffset"=w89, "PhoenixMotorControlDevRefIn"=w93) -> ("SetPosition"=w87:i32, "Success"=w92:bool)  [unwired: 4 in, 2 out]
          n40 = Bundle("WristOffset"=w89, "WristQuadPos"=w88, "SetPosition"=w87) -> (→"WristRecover":T29)  [unwired: 1 in]
        }
      }
      n41 = Compound Arithmetic op=AND(w60, w59, w58) -> (w57:bool)
      n42 = Bundle By Name(cluster=T27 {"ShoulderValid"=FALSE, "ExtensionValid"=FALSE, "WristValid"=FALSE} ("ArmPositionValidityOut"), "ShoulderValid"=w69, "ExtensionValid"=w68, "WristValid"=w67) -> (w56:T27)
      n43 = Cluster To Array(cluster=w56) -> (array=w55:bool[])
      n44 = And Array Elements(Boolean array=w55) -> (logical AND=w49:bool)
      n45 = Select(t=ArmHomingValidity."Valid", s=w49, f=w51) -> (s? t:f=w50:T25)
      n46 = Select(t=ArmHomingState."homing complete " ("ArmHomingStateIn"), s=w49, f=w52) -> (s? t:f=w53:T26)
    }
    frame True {
      # "All components valid.  No recovery necessary"
    }
  }
  "ArmPositionValidityOut" <- w19
  "ArmHomingStateOut" <- w10
  "ArmHomingValidityOut" <- w9
  "RecoveredOut" <- w15
  "ArmRecoveryParameters Out" <- "ArmRecoveryParameters In"
